vi "FPGA Main.vi"() -> ()   [LabVIEW 2015]
uses:
  <userlib>/_NI SPI IP/FPGA/Controllers/Public/Transfer Settings.ctl
  vi.lib/SPI API/Controls/SPI Digital IO Enable Lines.ctl
  <vilib>/Platform/TimedLoop/XDataNode/timing_clust.ctl
  <vilib>/Platform/TimedLoop/XDataNode/nitl_modes.ctl
  <vilib>/Platform/TimedLoop/XDataNode/wakeup.ctl
  vi.lib/SPI API/Controls/SPI Digital IO Lines.ctl
  <vilib>/rvi/Emulation/niFpgaGetClockAttributes.vi
  <vilib>/rvi/Emulation/niFpgaSctlEmulationGetInTimedLoop.vi
  <vilib>/rvi/Emulation/niFpgaEmulationReportErrorSimple.vi
  vi.lib/SPI API/Polymorphic VI Instances/Initialize SPI Engine Resources 128-bit.vi
  vi.lib/SPI API/Polymorphic VI Instances/Is SPI Engine Ready for Next Transaction 128-bit.vi
  <vilib>/rvi/Emulation/niFpgaCriticalErrorInLSC.vi
  vi.lib/SPI API/Polymorphic VI Instances/Set Data to Write for SPI Transaction 128-bit.vi
  vi.lib/SPI API/Polymorphic VI Instances/Set Full SPI Engine Configuration 128-bit.vi
  vi.lib/SPI API/Polymorphic VI Instances/Start SPI Transaction 128-bit.vi
  vi.lib/SPI API/Polymorphic VI Instances/Read SPI Response for SPI Transactions 128-bit.vi
  vi.lib/SPI API/Polymorphic VI Instances/SPI Engine 128-bit.vi
  <vilib>/Platform/TimedLoop/XDataNode/XDataNode.xnode
  vi.lib/SPI API/SPI API.lvlib
  <vilib>/Platform/TimedLoop/XDataNode/XDNodeRunTimeDep.lvlib
  <userlib>/_NI SPI IP/FPGA/Controllers/NI SPI IP FPGA.lvlib
panel:
  out "Data 8":u64=2147483648
  out "Data 7":u64=2147483648
  out "Data 6":u64=2147483648
  out "Data 5":u64=2147483648
  in  "Data 4":u64=2147483648
  in  "Data 3":u64=2147483648
  in  "Data 2":u64=2147483648
  in  "Data 1":u64=2147483648
  out "CS":bool
  out "SCLK":bool
  out "MOSI":bool
  in  "Chip Select":u8
  in  "SPI Physical Settings":T1={"Divide Value"=20, "Transfer Length (bits)"=32, "CS Asserted Polarity"=FALSE, "Clock Polarity (CPOL)"=FALSE, "Clock Phase (CPHA)"=FALSE, "Lengthen MISO Setup"=FALSE, "Direction Change Bit"=0, "MOSI Starts as Output"=FALSE, "Tristatable MOSI"=FALSE} {"Direction Change Bit" max=64 step=1; "Transfer Length (bits)" min=1 max=64 step=1}
  out "read Iterations":i32
  in  "Data To Write":u64=2147483648
  out "Slave Response":u64
  out "oclk div":u32
  out "oclk freq":u32
  in  "Sample Rate (S/s)":u32=10000
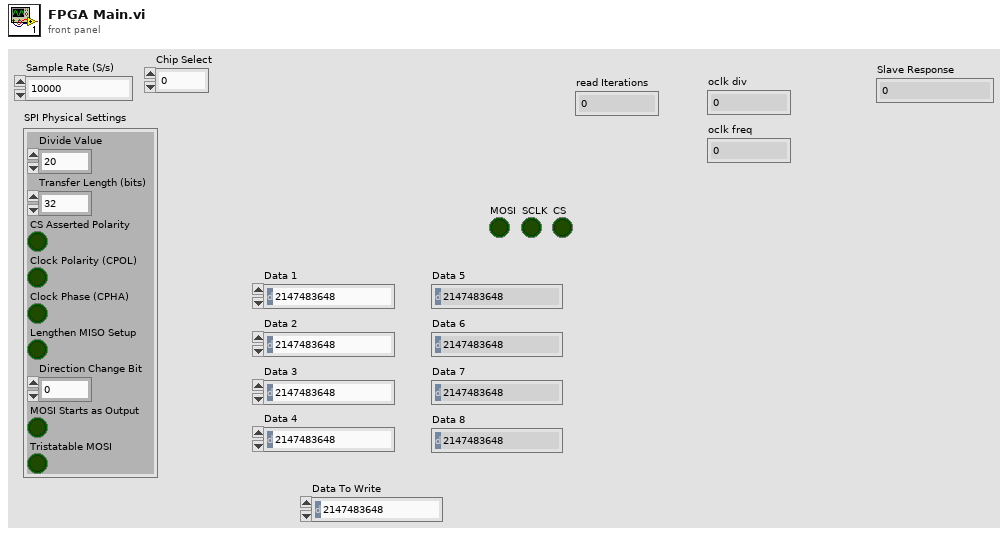
[diagram p1: front panel]
types:
  T1 = typedef "NI SPI IP FPGA.lvlib/Transfer Settings.ctl" = cluster{"Divide Value":u8, "Transfer Length (bits)":u8, "CS Asserted Polarity":bool, "Clock Polarity (CPOL)":bool, "Clock Phase (CPHA)":bool, "Lengthen MISO Setup":bool, "Direction Change Bit":u8, "MOSI Starts as Output":bool, "Tristatable MOSI":bool}
  T2 = typedef "SPI API.lvlib/SPI Digital IO Lines.ctl" = cluster{"SCLK":refnum<k21>, "MISO":refnum<k21>, "MOSI":refnum<k21>, "CS 0":refnum<k21>, "CS 1":refnum<k21>, "CS 2":refnum<k21>, "CS 3":refnum<k21>, "CS 4":refnum<k21>, "CS 5":refnum<k21>}
  T3 = typedef "SPI API.lvlib/SPI Digital IO Enable Lines.ctl" = cluster{"SCLK_en":refnum<k21>, "MISO_en":refnum<k21>, "MOSI_en":refnum<k21>, "CS0_en":refnum<k21>, "CS1_en":refnum<k21>, "CS2_en":refnum<k21>, "CS3_en":refnum<k21>, "CS4_en":refnum<k21>, "CS5_en":refnum<k21>}
  T4 = typedef "SPI API.lvlib/SPI Engine Resources 64-bit.ctl" = cluster{"To SPI Engine Data FIFO":refnum<k21>, "From SPI Engine Data FIFO":refnum<k21>, "Data to SPI Engine Cache Register":refnum<k21>, "SPI Transaction Settings Cache Register":refnum<k21>}
  T5 = typedef "SPI API.lvlib/SPI Engine Resources 128-bit.ctl" = cluster{"To SPI Engine Data FIFO":refnum<k21>, "From SPI Engine Data FIFO":refnum<k21>, "Data to SPI Engine Cache Register":refnum<k21>, "SPI Transaction Settings Cache Register":refnum<k21>}
  T6 = typedef "XDNodeRunTimeDep.lvlib/timing_clust.ctl" = cluster{"Expected End [f-1]":u64, "Actual End [f-1]":u64, "Finished Late? [f-1]":bool, "Expected End [i-1]":u64, "Actual End [i-1]":u64, "Finished Late? [i-1]":bool, "Expected Start [i]":u64, "Actual Start [i]":u64, "Expected Start [f]":u64, "Actual Start [f]":u64, "Source Name":string, "Structure Name":string, "Period":i64, "Deadline":i64, "Offset":i64, "Start":i64, "Priority":i32, "Timeout":i32, "Mode":T7, "Wakeup Reason":T8, "Error":errorcluster, "Source Type":string, "Secondary Source Type":string, "Global End Time":u64, "Global Start Time":u64, "Frame Duration":u64, "Iteration Duration":u64, "Assigned CPU":i32, "I/O Scan Engine Mode":u32}
  T7 = typedef "XDNodeRunTimeDep.lvlib/nitl_modes.ctl" = enum32{"No Change", "Process missed periods, maintain original phase", "Discard missed periods, maintain original phase", "Process missed periods, ignore original phase", "Discard missed periods, ignore original phase"}
  T8 = typedef "XDNodeRunTimeDep.lvlib/wakeup.ctl" = enum32{"Normal", "Aborted", "Asynchronous wakeup", "Timing source error", "Timed loop error", "Timeout"}
  T9 = typedef "SPI API.lvlib/SPI API Response Data 128-bit.ctl" = cluster{"Response Data":T10, "Node Id":u16}
  T10 = typedef "SPI API.lvlib/SPI API Data 128-bit.ctl" = bool[]
  T11 = typedef "NI SPI IP FPGA.lvlib/Spi Master Inputs.ctl" = cluster{"MISO":bool}
  T12 = typedef "NI SPI IP FPGA.lvlib/Spi Master Outputs.ctl" = cluster{"Chip Select":bool, "Clock":bool, "MOSI":bool, "MOSI OE":bool}
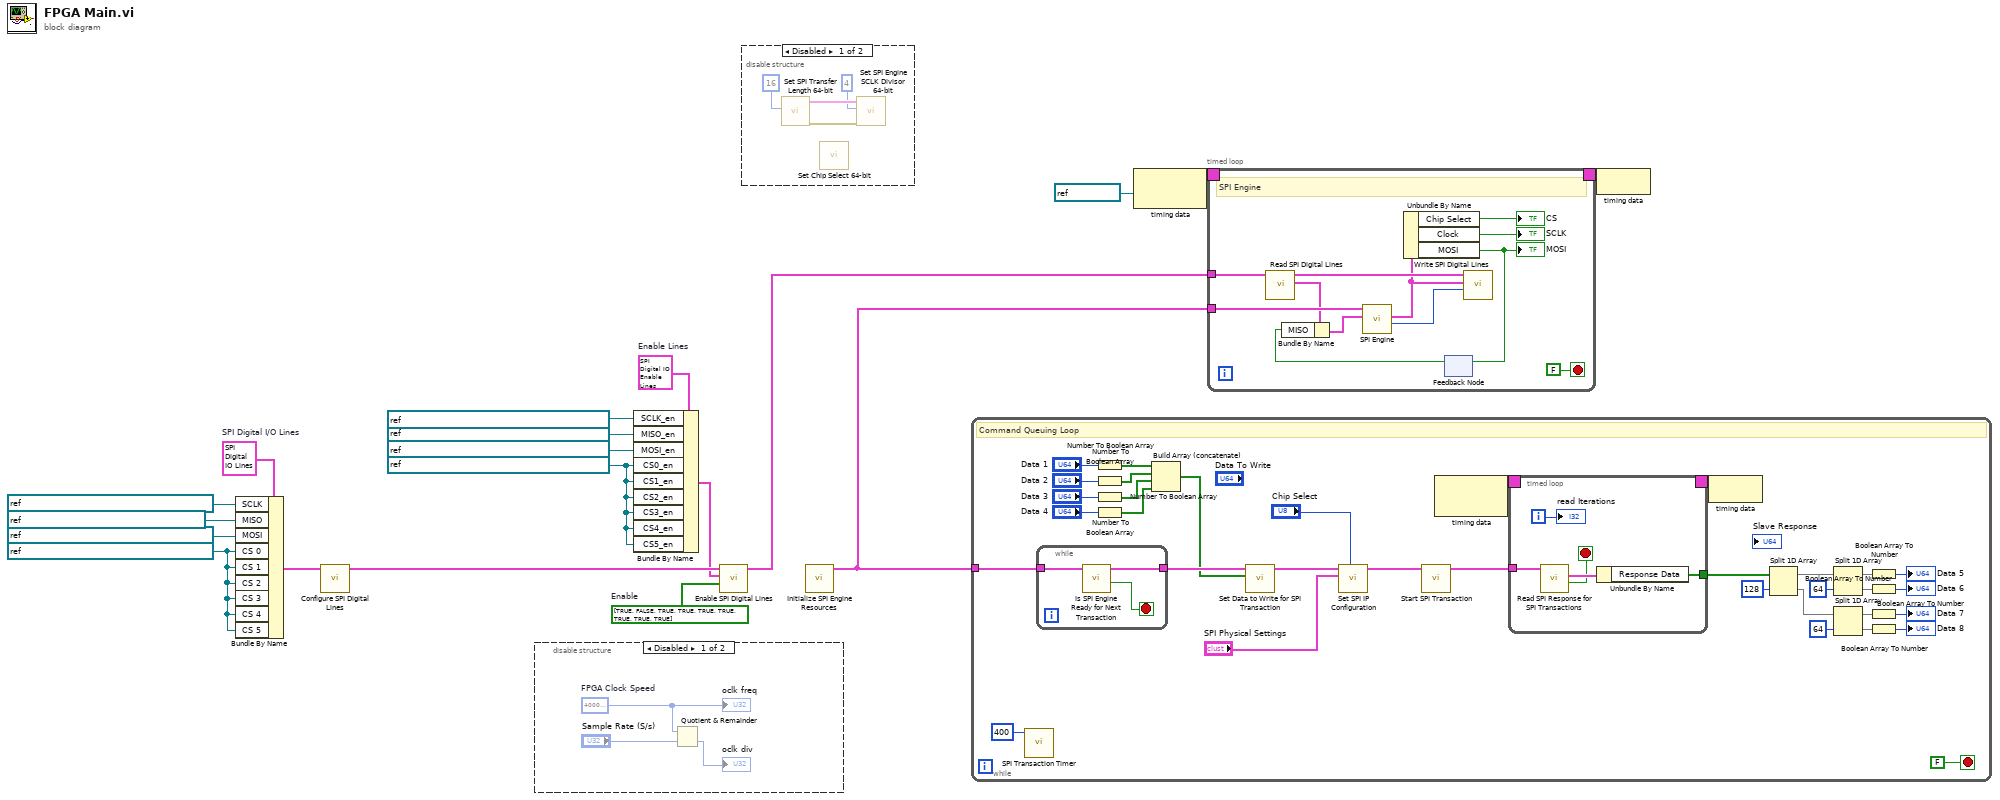
[diagram p0: block diagram]
diagram:
  w4 = refnum<k21> "sbRIO-9651 Socket\\PMOD1_Pin1_enable" ("CS0_en")
  w5 = refnum<k21> "sbRIO-9651 Socket\\PMOD1_Pin1_out" ("CS 0")
  w14 = T2 {"SCLK"="sbRIO-9651 Socket\\PMOD1_Pin4_out", "MISO"="sbRIO-9651 Socket\\PMOD1_Pin3_in", "MOSI"="sbRIO-9651 Socket\\PMOD1_Pin2_out", "CS 0"="sbRIO-9651 Socket\\PMOD1_Pin1_out", "CS 1"="sbRIO-9651 Socket\\PMOD1_Pin1_out", "CS 2"="sbRIO-9651 Socket\\PMOD1_Pin1_out", "CS 3"="sbRIO-9651 Socket\\PMOD1_Pin1_out", "CS 4"="sbRIO-9651 Socket\\PMOD1_Pin1_out", "CS 5"="sbRIO-9651 Socket\\PMOD1_Pin1_out"}  # SPI Digital I/O Lines
  w2 = bool[] [TRUE, FALSE, TRUE, TRUE, TRUE, TRUE, TRUE, TRUE, TRUE]  # Enable
  w9 = T3 {"SCLK_en"="sbRIO-9651 Socket\\PMOD1_Pin4_enable", "MISO_en"="sbRIO-9651 Socket\\PMOD1_Pin3_enable", "MOSI_en"="sbRIO-9651 Socket\\PMOD1_Pin2_enable", "CS0_en"="sbRIO-9651 Socket\\PMOD1_Pin1_enable", "CS1_en"="sbRIO-9651 Socket\\PMOD1_Pin1_enable", "CS2_en"="sbRIO-9651 Socket\\PMOD1_Pin1_enable", "CS3_en"="sbRIO-9651 Socket\\PMOD1_Pin1_enable", "CS4_en"="sbRIO-9651 Socket\\PMOD1_Pin1_enable", "CS5_en"="sbRIO-9651 Socket\\PMOD1_Pin1_enable"}  # Enable Lines
  n1 = Bundle By Name(cluster=w14, "SCLK"=refnum<k21> "sbRIO-9651 Socket\\PMOD1_Pin4_out", "MISO"=refnum<k21> "sbRIO-9651 Socket\\PMOD1_Pin3_in", "MOSI"=refnum<k21> "sbRIO-9651 Socket\\PMOD1_Pin2_out", "CS 0"=w5, "CS 1"=w5, "CS 2"=w5, "CS 3"=w5, "CS 4"=w5, "CS 5"=w5) -> (w10:T2)
  n2 = call "Configure SPI Digital Lines.vi"("SPI Digital I/O Lines"=w10) -> ("SPI Digital I/O Lines"=w16:T2)  [unwired: 9 in, 1 out]
  n3 = disable-structure shown="Disabled" {
    frame Disabled {
      w20 = u32 40000000  # FPGA Clock Speed
      n4 = Quotient & Remainder(x=w20, y="Sample Rate (S/s)") -> (x-y*floor(x/y)=w23:u32, floor(x/y)=→"oclk div":u32)
      "oclk freq" <- w20
    }
    frame Enabled {
    }
  }
  n5 = Bundle By Name(cluster=w9, "SCLK_en"=refnum<k21> "sbRIO-9651 Socket\\PMOD1_Pin4_enable", "MISO_en"=refnum<k21> "sbRIO-9651 Socket\\PMOD1_Pin3_enable", "MOSI_en"=refnum<k21> "sbRIO-9651 Socket\\PMOD1_Pin2_enable", "CS0_en"=w4, "CS1_en"=w4, "CS2_en"=w4, "CS3_en"=w4, "CS4_en"=w4, "CS5_en"=w4) -> (w3:T3)
  n6 = call "Enable SPI Digital Lines.vi"("Enable Lines States"=w2, "Enable Lines"=w3, "SPI Digital I/O Lines"=w16) -> ("SPI Digital I/O Lines"=w15:T2)  [unwired: 7 in, 1 out]
  n7 = disable-structure shown="Disabled" {
    frame Disabled {
      n8 = call "Set SPI Transfer Length 64-bit.vi"("Transfer Length (bits)"=u8 16) -> ("error out"=w27:errorcluster, "SPI Engine Resources"=w26:T4)  [unwired: 9 in]
      n9 = call "Set Chip Select 64-bit.vi"() -> ()  [unwired: 10 in, 2 out]
      n10 = call "Set SPI Engine SCLK Divisor 64-bit.vi"("error in"=w27, "SPI Engine Clock Divisor"=u8 4, "SPI Engine Resources"=w26) -> ()  [unwired: 6 in, 3 out]
    }
    frame Enabled {
    }
  }
  n11 = call-poly "Initialize SPI Engine Resources.vi"() -> ("SPI Engine Resources 128-bit"=w1:T5)  [unwired: 10 in, 1 out]
  n12 = while {
    tunnel: w1 -> [w61]
    stop <- FALSE stop-if-true
    # "Command Queuing Loop"
    n13 = call "SPI Transaction Timer.vi"("Loop Time (Ticks)"=u32 400) -> ()  [unwired: 10 in, 1 out]
    n14 = while {
      tunnel: w61 -> [w64]
      tunnel: [w63] -> w56
      stop <- w62 stop-if-true
      n15 = call-poly "Is SPI Engine Ready for Next Transaction.vi"("SPI Engine Resources"=w64) -> ("SPI Engine Ready?"=w62:bool, "SPI Engine Resources"=w63:T5)  [unwired: 7 in, 2 out]
    }
    n16 = Number To Boolean Array(number="Data 1") -> (Boolean array=w47:bool[])
    n17 = Number To Boolean Array(number="Data 2") -> (Boolean array=w48:bool[])
    n18 = Number To Boolean Array(number="Data 3") -> (Boolean array=w34:bool[])
    n19 = Number To Boolean Array(number="Data 4") -> (Boolean array=w33:bool[])
    n20 = Build Array (concatenate)(w47, w48, w34, w33) -> (w32:bool[])
    n21 = call-poly "Set Data to Write for SPI Transaction.vi"("Data"=w32, "SPI Engine Resources"=w56) -> ("SPI Engine Resources"=w55:T5)  [unwired: 8 in, 1 out]
    n22 = call-poly "Set SPI IP Configuration.vi"("Chip Select"="Chip Select", "SPI Physical Settings"="SPI Physical Settings", "SPI Engine Resources"=w55) -> ("SPI Engine Resources"=w52:T5)  [unwired: 7 in, 1 out]
    n23 = call-poly "Start SPI Transaction.vi"("SPI Engine Resources 2"=w52) -> ("SPI Engine Resources"=w51:T5)  [unwired: 8 in, 2 out]
    n24 = node-c288() -> (w60:T6)  [unwired: 1 in]
    n25 = timed-loop {
      timing: w60 -> [_]
      timing-out: [_] -> w59
      tunnel: w51 -> [w68]
      tunnel: [w65] -> w45
      i -> [w69]
      stop <- w66 stop-if-true
      n26 = call-poly "Read SPI Response for SPI Transactions.vi"("SPI Engine Resources"=w68) -> ("Read Data Valid?"=w66:bool, "Read Data"=w67:T9)  [unwired: 7 in, 2 out]
      n27 = Unbundle By Name(w67) -> ("Response Data"=w65:T10)
      "read Iterations" <- w69
    }
    n28 = node-c288(w59) -> ()
    n29 = Split 1D Array(array=w45, index=128) -> (first subarray=w44:T10, second subarray=w43:T10)
    n30 = Split 1D Array(array=w44, index=64) -> (first subarray=w40:T10, second subarray=w39:T10)
    n31 = Split 1D Array(array=w43, index=64) -> (first subarray=w38:T10, second subarray=w37:T10)
    n32 = Boolean Array To Number(Boolean array=w40) -> (number=→"Data 5":u64)
    n33 = Boolean Array To Number(Boolean array=w39) -> (number=→"Data 6":u64)
    n34 = Boolean Array To Number(Boolean array=w38) -> (number=→"Data 7":u64)
    n35 = Boolean Array To Number(Boolean array=w37) -> (number=→"Data 8":u64)
  }
  n36 = node-c288(refnum<k21> "120MHz" ("Source Name")) -> (w19:T6)
  n37 = timed-loop {
    tunnel: w1 -> [w82]
    tunnel: w15 -> [w84]
    timing: w19 -> [_]
    timing-out: [_] -> w18
    stop <- FALSE stop-if-true
    # "SPI Engine"
    n38 = call "Read SPI Digital Lines.vi"("SPI Digital I/O Lines"=w84) -> ("SPI Read Data"=w79:T11, "SPI Digital I/O Lines"=w83:T2)  [unwired: 8 in, 1 out]
    n39 = feedback #1() -> (w76:bool)  [unwired: 1 in]
    n40 = Bundle By Name(cluster=w79, "MISO"=w76) -> (w78:T11)
    n41 = call-poly "SPI Engine.vi"("SPI Read Data"=w78, "SPI Engine Resources"=w82) -> ("Chip Select"=w81:u8, "SPI Write Data"=w80:T12)  [unwired: 6 in, 2 out]
    n42 = Unbundle By Name(w80) -> ("Chip Select"=→"CS":bool, "Clock"=→"SCLK":bool, "MOSI"=w77:bool)
    "MOSI" <- w77
    n43 = feedback-in #1(w77) -> ()
    n44 = call "Write SPI Digital Lines.vi"("Chip Select"=w81, "SPI Write Data"=w80, "SPI Digital I/O Lines"=w83) -> ()  [unwired: 7 in, 2 out]
  }
  n45 = node-c288(w18) -> ()
